vi "Queue add.vi"(8 "Queue B in":T1, 10 "Message Cluster":T2) -> ()   [LabVIEW 2015]
uses:
  QMH Fundamentals - Message Cluster.ctl
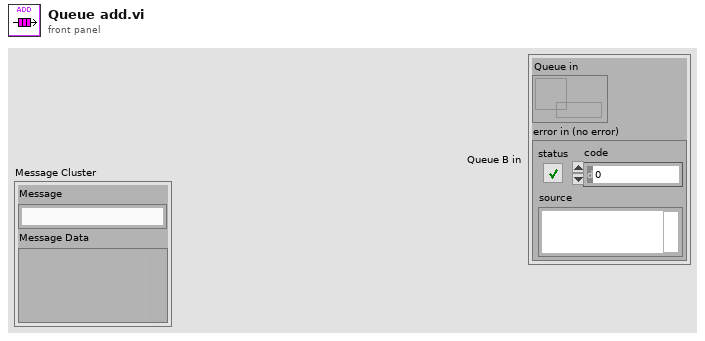
[diagram p1: front panel]
types:
  T1 = cluster{"Queue in":refnum<queue>, "error in (no error)":errorcluster}
  T2 = typedef "QMH Fundamentals - Message Cluster.ctl" = cluster{"Message":string, "Message Data":variant}
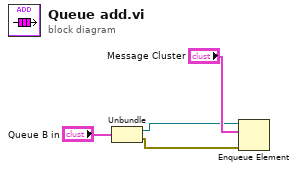
[diagram p0: block diagram]
diagram:
  n1 = Unbundle("Queue B in") -> ("Queue in"=w2:refnum<queue>, "error in (no error)"=w1:errorcluster)
  n2 = Enqueue Element(queue=w2, element="Message Cluster", error in (no error)=w1) -> ()  [unwired: 1 in, 3 out]
